vi "Fire Stop User Event.vi"(8 "error in (no error)":errorcluster, 11 "Wait User Events":T1) -> (0 "error out":errorcluster)   [LabVIEW 2023, in "Weather Wait Loop.lvlib"]
doc: "Generates the wait message loop's stop user event to notify the event loop to exit."
uses:
  Weather Wait Loop.lvlib
  User Events.ctl
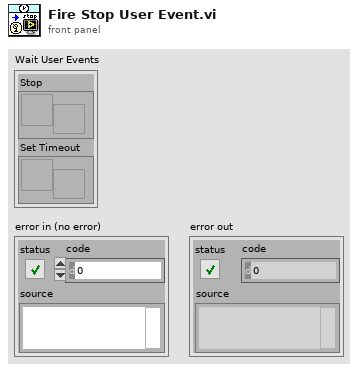
[diagram p1: front panel]
types:
  T1 = typedef "Weather Wait Loop.lvlib/User Events.ctl" = cluster{"Stop":refnum<user-event>, "Set Timeout":refnum<user-event>}
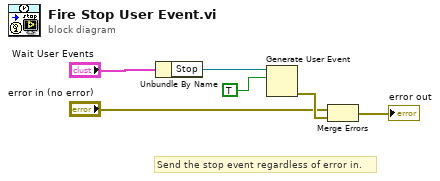
[diagram p0: block diagram]
diagram:
  # "Send the stop event regardless of error in."
  n1 = Unbundle By Name("Wait User Events") -> ("Stop"=w4:refnum<user-event>)
  n2 = Generate User Event(user event=w4, event data cluster=TRUE ("event data")) -> (error out=w6:errorcluster)  [unwired: 2 in, 1 out]
  n3 = Merge Errors("error in (no error)", w6) -> (→"error out":errorcluster)
